vi "Untitled 1.vi"() -> ()   [LabVIEW 2022 SP3]
panel:
  in  "Text":string
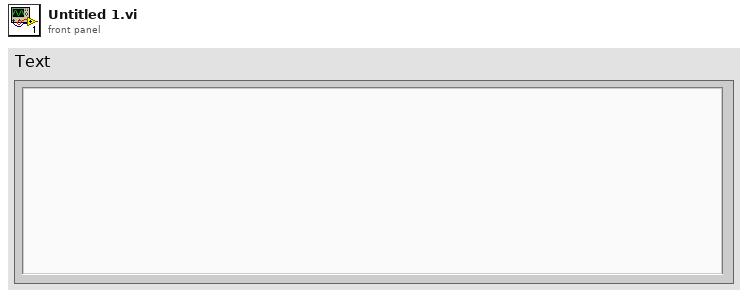
[diagram p1: front panel]
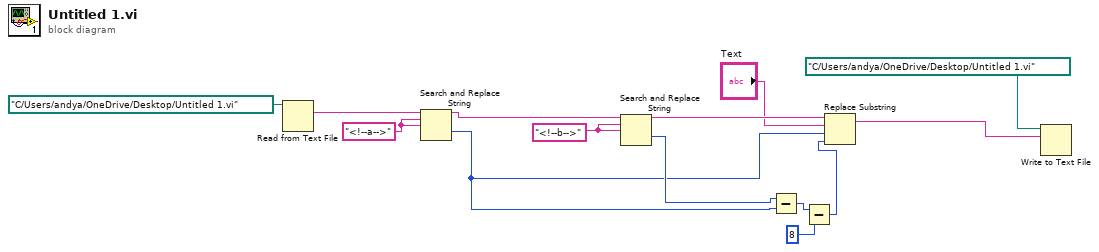
[diagram p0: block diagram]
diagram:
  w10 = "<!--b-->" ("search string")
  w12 = "<!--a-->" ("search string")
  n1 = Read from Text File(file (use dialog)=path "C:/Users/andya/OneDrive/Desktop/Untitled 1.vi") -> (text=w13:string)  [unwired: 3 in, 3 out]
  n2 = Search and Replace String(input string=w13, search string=w12, replace string=w12) -> (result string=w11:string, offset past replacement=w7:i32)  [unwired: 5 in, 2 out]
  n3 = Search and Replace String(input string=w11, search string=w10, replace string=w10) -> (result string=w9:string, offset past replacement=w8:i32)  [unwired: 5 in, 2 out]
  n4 = Subtract(x=w8, y=w7) -> (x-y=w4:i32)
  n5 = Subtract(x=w4, y=8) -> (x-y=w2:i32)
  n6 = Replace Substring(2:w2, 3:w7, 4:"Text", 5:w9) -> (1:w5:string)  [unwired: 1 out]
  n7 = Write to Text File(file (use dialog)=path "C:/Users/andya/OneDrive/Desktop/Untitled 1.vi", text=w5) -> ()  [unwired: 2 in, 3 out]
